vi "Search ColorCenter.vi"() -> ()   [LabVIEW 2020]
uses:
  Labview Library/Libraries/Color Center Repository/Libraries/Repository Control/Map Element.ctl
  Labview Library/Libraries/Color Center Repository/Libraries/Repository Control/Repository Control.lvlib
panel:
  out "All Possible ColorCenter":T1[](array[typedef])
  out "Nearest Distance":dbl
  out "Nearest ColorCenter":T1
  in  "Distance Threshold(um)":dbl=0.2 format="%#_13g"
  in  "Map":T1[](array[typedef])
  in  "Position":dbl[](array[numeric])
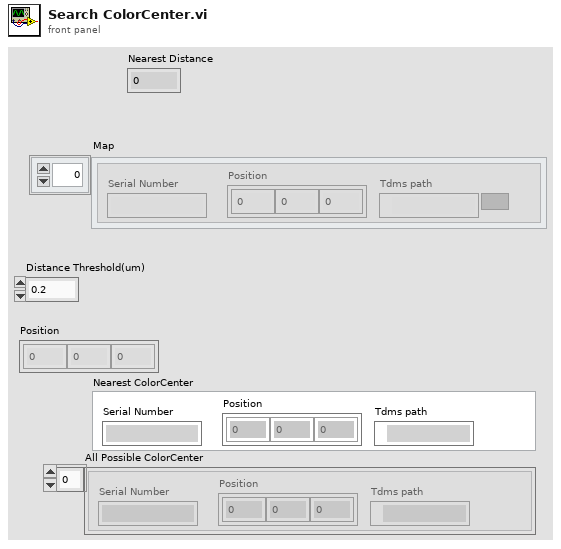
[diagram p1: front panel]
types:
  T1 = typedef "Repository Control.lvlib/Map Element.ctl" = cluster{"Position":dbl[], "Serial Number":string, "Tdms path":path}
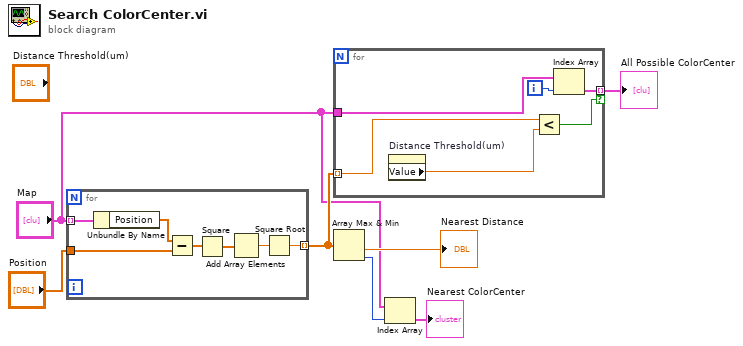
[diagram p0: block diagram]
diagram:
  n1 = for {
    tunnel: "Map" -> [w14] mode=indexing
    tunnel: "Position" -> [w12]
    tunnel: [w8] -> w3 mode=indexing
    n2 = Unbundle By Name(w14) -> ("Position"=w13:dbl[])
    n3 = Subtract(x=w13, y=w12) -> (x-y=w11:dbl[])
    n4 = Square(x=w11) -> (x^2=w10:dbl[])
    n5 = Add Array Elements(numeric array=w10) -> (sum=w9:dbl)
    n6 = Square Root(x=w9) -> (sqrt(x)=w8:dbl)
  }
  n7 = for {
    tunnel: w3 -> [w20] mode=indexing
    tunnel: [w16] -> w1 mode=indexing if=w19
    tunnel: "Map" -> [w17]
    i -> [w18]
    n8 = property on="Distance Threshold(um)" class="DigNum (strict)"() -> ("Value"=w15:dbl)  [unwired: 2 in, 2 out]
    n9 = Less?(x=w20, y=w15) -> (x < y?=w19:bool)
    n10 = Index Array(array=w17, index=w18) -> (element=w16:T1)
  }
  "All Possible ColorCenter" <- w1
  n11 = Array Max & Min(array=w3) -> (min value=→"Nearest Distance":dbl, min index (indices)=w6:i32)  [unwired: 2 out]
  n12 = Index Array(array="Map", index=w6) -> (element=→"Nearest ColorCenter":T1)
